vi "DB_GetModule.vi"(8 "error in (no error)":errorcluster) -> (0 "error out":errorcluster, 3 "Data":string[](array[string]))   [LabVIEW 2015, in "Settings-Style.lvlib"]
uses:
  Settings-Style.lvlib
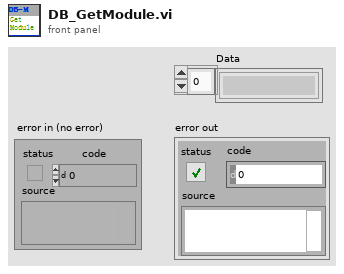
[diagram p1: front panel]
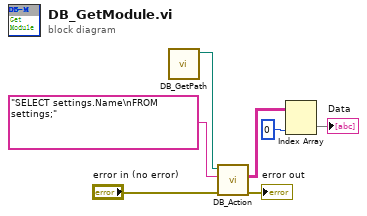
[diagram p0: block diagram]
diagram:
  n1 = call "DB_GetPath.vi"() -> ("appended path"=w1:path)  [unwired: 11 in]
  n2 = call "DB_Action.vi"("error in"="error in (no error)", "Command Text"="SELECT settings.Name\nFROM settings;", "路径"=w1) -> ("error out"=→"error out":errorcluster, "Data"=w6:string[][])  [unwired: 7 in]
  n3 = Index Array(array=w6, index (col)=0 ("disabled index (col)")) -> (element=→"Data":string[])  [unwired: 1 in]
